vi "MCL Get Handle By Serial.vi"(8 "error in (no error)":errorcluster, 11 "serial":i16) -> (0 "error out":errorcluster, 3 "function return":i32)   [LabVIEW 2014, in "Madlib.lvlib"]
doc: "MADLIB_API int MCL_GetHandleBySerial(short serial);"
uses:
  <userlib>/Lambda2/lib/Madlib/Madlib.lvlib
  <userlib>/Lambda2/lib/Madlib/Madlib.dll
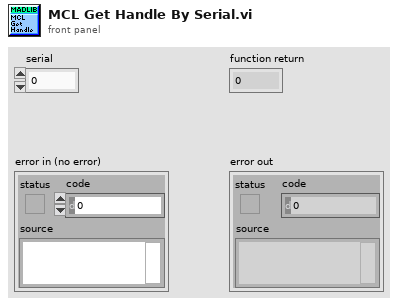
[diagram p1: front panel]
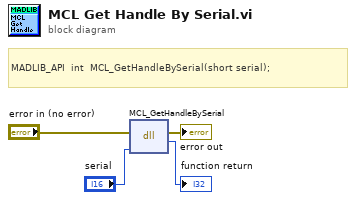
[diagram p0: block diagram]
diagram:
  # "MADLIB_API  int\t\tMCL_GetHandleBySerial(short serial);"
  n1 = dll-call lib="C:/Program Files (x86)/National Instruments/LabVIEW 2014/user.lib/Lambda2/lib/Madlib/Madlib.*" fn="MCL_GetHandleBySerial"(error in="error in (no error)", "serial"="serial") -> (error out=→"error out":errorcluster, →"function return":i32)  [unwired: 3 in, 1 out]
